vi "Get Value.vi"(8 "error in (no error)":errorcluster, 11 "Filled Text Fields in":refnum<class "Filled Text Fields.lvclass">) -> (0 "error out":errorcluster, 2 "Value":string, 3 "Filled Text Fields out":refnum<class "Filled Text Fields.lvclass">)   [LabVIEW 2017, in "Filled Text Fields.lvlib" / "Filled Text Fields.lvclass"]
uses:
  Filled Text Fields.lvclass
  Filled Text Fields.lvclass/Filled Text Fields.ctl
  Data/Data.lvclass/Data.ctl
  Data/getData.vi
  Data/Data.lvclass
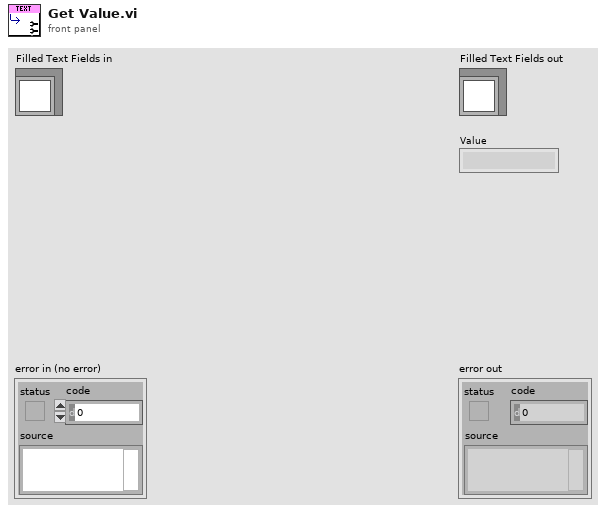
[diagram p1: front panel]
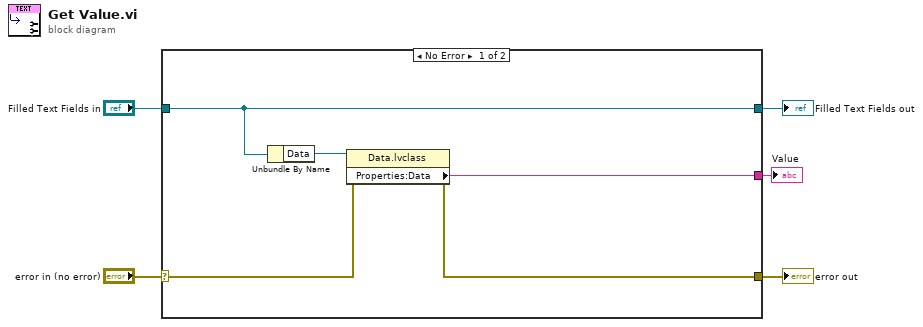
[diagram p0: block diagram]
diagram:
  n1 = case shown="No Error" "error in (no error)" {
    selector: "error in (no error)" -> [w7 w12]
    tunnel: [w6 w12] -> w4
    tunnel: [w10 w11] -> w2
    tunnel: "Filled Text Fields in" -> [w10 w11]
    tunnel: [w8 _] -> w1
    frame No Error {
      n2 = Unbundle By Name(w10) -> ("Data"=w9:refnum<class "Data.lvclass">)
      n3 = property class="Data.lvclass"(reference=w9, error in=w7) -> (error out=w6:errorcluster, "Properties:Data"=w8:string)  [unwired: 1 out]
    }
    frame Error {
    }
  }
  "error out" <- w4
  "Filled Text Fields out" <- w2
  "Value" <- w1
